vi "HEWH Adjust Temp Flow.vi"(0 "Core HEWH Data Station A":T2 {"Test Patten Setup"."PRAT/RLT Sequence"."Time" format="%<%H:%M:%S>t"; "Test Patten Setup"."Total Gallons Schedule" format="%.2f"}, 1 "MW100 Input":refnum<visa-resource-name>, 2 "Disable Temp Adjust?":bool, 3 "MW100 Sema":T18, 4 "GPM Target":T19 format="%.2f", 5 "error in (no error)":errorcluster, 6 "Elapsed Time (sec)":dbl, 7 "Temperature":T19 format="%.2f", 8 "State":T1, 10 "PID gains (Temp)":T20={"proportional gain (Kc)"=0.1, "integral time (Ti, min)"=0.01, "derivative time (Td, min)"=0.0} {"derivative time (Td, min)" format="%.3f"; "integral time (Ti, min)" format="%.3f"; "proportional gain (Kc)" format="%.3f"}, 11 "Debug":bool, 12 "Adjust Temp Timer":dbl=1.0 format="%#_13g", 13 "Use Fuzzy Logic":bool) -> (14 "Core HEWH Data out":T2 {"Test Patten Setup"."PRAT/RLT Sequence"."Time" format="%<%H:%M:%S>t"; "Test Patten Setup"."Total Gallons Schedule" format="%.2f"}, 15 "MW100 Output":refnum<visa-resource-name>, 18 "Adjusting Temp":bool, 19 "error out":errorcluster)   [LabVIEW 2016]
uses:
  Utility/Custom Pallet Controls/Custom Pallet DBL.ctl
  Type Definitions/HEWH Output Information.ctl
  Type Definitions/HEWH Draw Pattern Setup.ctl
  Type Definitions/PRAT Test.ctl
  Utility/Save File/File Setup (Public)/Type Definition/Save File HEWH Heating Control Mode.ctl
  Type Definitions/Terminate Draw Conditions.ctl
  Type Definitions/HEWH Start Conditions.ctl
  Type Definitions/Check Special Condtions.ctl
  Type Definitions/HEWH Special Condition Check.ctl
  Type Definitions/HEWH Draw Flag ENUM.ctl
  Type Definitions/HEWH Specific DAQ.ctl
  Type Definitions/HEWH Power Data.ctl
  Type Definitions/HEWH Power Elements.ctl
  Utility/Type Definitions/UTILITY Power Analyzer.ctl
  Type Definitions/HEWH Calc and Calibration.ctl
  Utility/Save File/File Setup (Public)/Type Definition/Save File DOE LabView Program.ctl
  Custom Instrument Control/MW100/Type Definitions/Station ID Selector.ctl
  Type Definitions/HEWH Purge Draw.ctl
  Utility/Save File/File Setup.lvlib
panel:
  out "uA Output Flow":i32
  out "uA Output Temp":i32
  # "Draw Pattern Setup (24 Hour)"
  # "Draw Pattern Setup (24 Hour)"
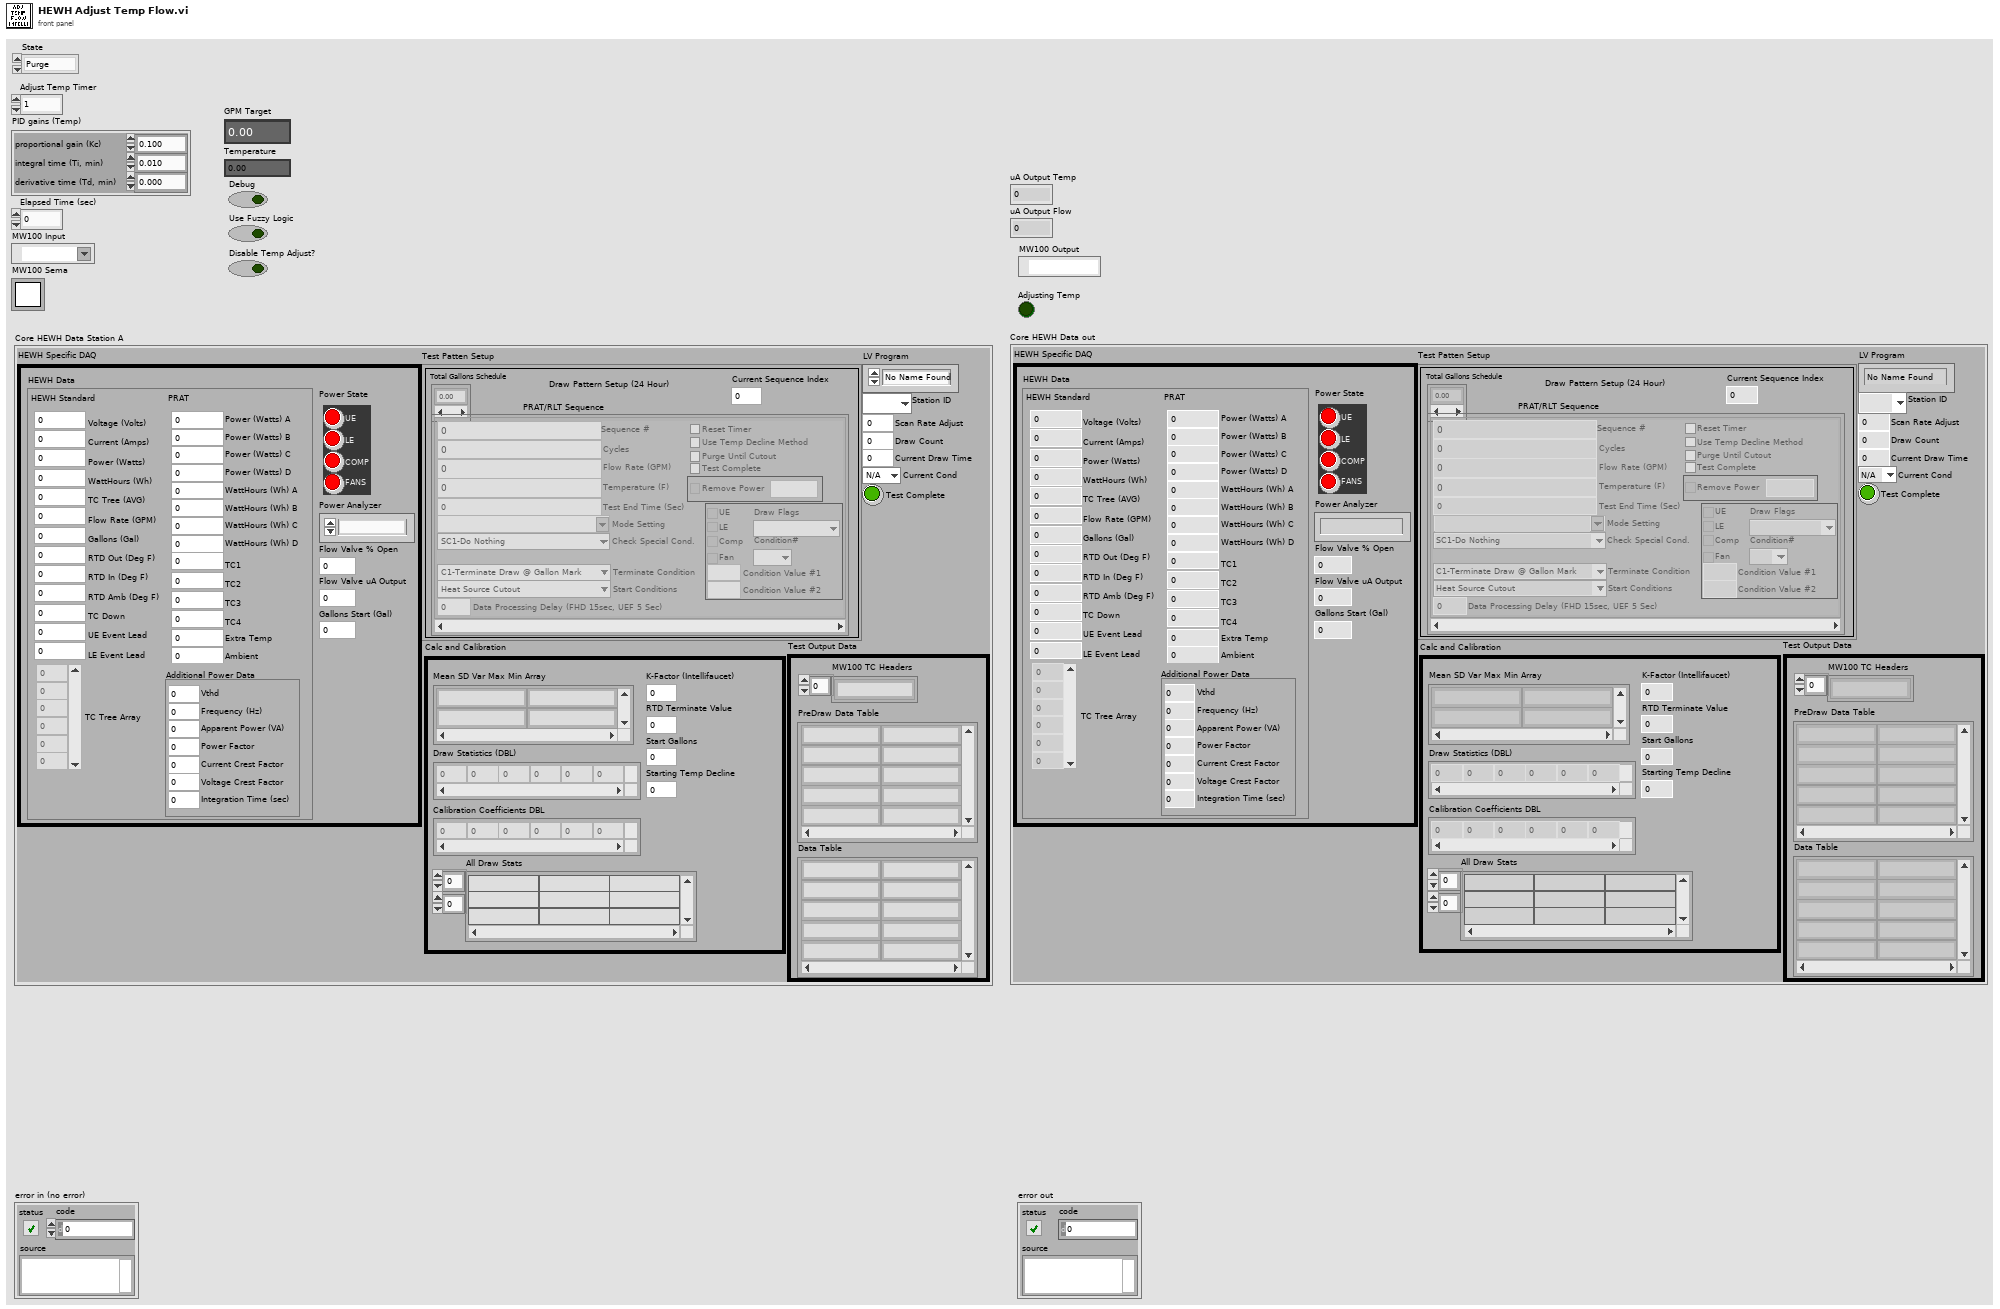
[diagram p1: front panel]
types:
  T1 = typedef "HEWH Purge Draw.ctl" = enum16{"Purge", "Draw"}
  T2 = typedef "HEWH Output Information.ctl" = cluster{"Scan Rate Adjust":dbl, "Draw Count":i32, "Test Patten Setup":T3, "HEWH Specific DAQ":T11, "Test Output Data":cluster{"PreDraw Data Table":string[][], "Data Table":string[][], "MW100 TC Headers":string[]}, "Calc and Calibration":T15, "Current Draw Time":dbl, "LV Program":T16, "Station ID":T17, "Current Cond":T9, "Test Complete":bool}
  T3 = typedef "HEWH Draw Pattern Setup.ctl" = cluster{"Total Gallons Schedule":dbl[], "PRAT/RLT Sequence":T4[], "Current Sequence Index":i32}
  T4 = typedef "PRAT Test.ctl" = cluster{"Sequence #":dbl, "Cycles":i32, "Mode Setting":T5, "Flow Rate (GPM)":dbl, "Temperature (F)":dbl, "Reset Timer":bool, "Use Temp Decline Method":bool, "Terminate Condition":T6, "Condition Value #1":dbl, "UE":bool, "LE":bool, "Comp":bool, "Fan":bool, "Test End Time (Sec)":dbl, "Purge Until Cutout":bool, "Start Conditions":T7, "Condition Value #2":dbl, "Remove Power":bool, "Time":dbl, "Check Special Cond.":T8, "Condition#":T9, "Draw Flags":T10, "Data Processing Delay (FHD 15sec, UEF 5 Sec)":dbl, "Test Complete":bool}
  T5 = typedef "File Setup.lvlib/Save File HEWH Heating Control Mode.ctl" = string
  T6 = typedef "Terminate Draw Conditions.ctl" = enum16{"C1-Terminate Draw @ Gallon Mark", "C2-Special Last Draw (HU Test)", "C3-RTD Out <=", "C4-Mean Tank Temp <=", "C5-Decrease RTD Out (Deg F)", "C6-Time (Seconds)", "C7-Until Any Heat Source", "C8-Specific Heat Source", "C9-Do Nothing"}
  T7 = typedef "HEWH Start Conditions.ctl" = enum16{"Heat Source Cutout", "At Time (Seconds)", "Every X (Seconds)", "T2 >= X° Below Setpoint", "Seconds From Complete", "Wait for LE & Comp Cutout", "Wait for Comp Cutout", "Wait for LE Cutout", "Wait for UE Cutout"}
  T8 = typedef "Check Special Condtions.ctl" = enum16{"SC1-Do Nothing", "SC2-Check Heat Source (On-C2/Off-C1)", "SC3-Check Skip Condition", "SC4-Check Heat Source ON/Fail"}
  T9 = typedef "HEWH Special Condition Check.ctl" = enum16{"N/A", "C1", "C2", "Reset/Fail", "Skip Draw Sequence"}
  T10 = typedef "HEWH Draw Flag ENUM.ctl" = enum16{"N/A", "None(0)", "Sml(1)", "Med(2)", "SmlMed(3)", "Lrg(4)", "SmlLrg(5)", "MedLrg(6)", "SmlMedLrg(7)"}
  T11 = typedef "HEWH Specific DAQ.ctl" = cluster{"HEWH Data":T12, "Flow Valve % Open":dbl, "Power State":T13, "Power Analyzer":T14, "Flow Valve uA Output":i32, "Gallons Start (Gal)":dbl}
  T12 = typedef "HEWH Power Data.ctl" = cluster{"HEWH Standard":cluster{"Voltage (Volts)":dbl, "Current (Amps)":dbl, "Power (Watts)":dbl, "WattHours (Wh)":dbl, "TC Tree (AVG)":dbl, "Flow Rate (GPM)":dbl, "Gallons (Gal)":dbl, "RTD Out (Deg F)":dbl, "RTD In (Deg F)":dbl, "RTD Amb (Deg F)":dbl, "TC Down":dbl, "UE Event Lead":i32, "LE Event Lead":i32, "TC Tree Array":dbl[]}, "PRAT":cluster{"Power (Watts) A":dbl, "Power (Watts) B":dbl, "Power (Watts) C":dbl, "Power (Watts) D":dbl, "TC1":dbl, "TC2":dbl, "TC3":dbl, "TC4":dbl, "WattHours (Wh) A":dbl, "WattHours (Wh) B":dbl, "WattHours (Wh) C":dbl, "WattHours (Wh) D":dbl, "Ambient":dbl, "Extra Temp":dbl}, "Additional Power Data":cluster{"Vthd":dbl, "Frequency (Hz)":dbl, "Apparent Power (VA)":dbl, "Power Factor":dbl, "Current Crest Factor":dbl, "Voltage Crest Factor":dbl, "Integration Time (sec)":dbl}}
  T13 = typedef "HEWH Power Elements.ctl" = cluster{"UE":bool, "LE":bool, "COMP":bool, "FANS":bool}
  T14 = typedef "UTILITY Power Analyzer.ctl" = enum16{"", "APLUS", "WT210", "WT500", "WT300", "OSI", "Debug", "WT230", "WT300_1", "WT300_2"}
  T15 = typedef "HEWH Calc and Calibration.ctl" = cluster{"Mean SD Var Max Min Array":string[][], "Draw Statistics (DBL)":dbl[][], "Calibration Coefficients DBL":dbl[][], "Start Gallons":dbl, "Starting Temp Decline":dbl, "K-Factor (Intellifaucet)":dbl, "All Draw Stats":string[][], "RTD Terminate Value":dbl}
  T16 = typedef "File Setup.lvlib/Save File DOE LabView Program.ctl" = enum16{"No Name Found", "DOE Stand", "Dishwasher Kitchen", "Portable Stand", "HEWH", "Dryer", "Dryer WILT", "HCC", "PRAT", "HEWH RLT", "Refrigeration"}
  T17 = typedef "Station ID Selector.ctl" = enum16{"", "A", "B", "C", "D", "Global"}
  T18 = typedef "Semaphore RefNum" = refnum<k1>
  T19 = typedef "Custom Pallet DBL.ctl" = dbl
  T20 = cluster{"proportional gain (Kc)":dbl, "integral time (Ti, min)":dbl, "derivative time (Td, min)":dbl}
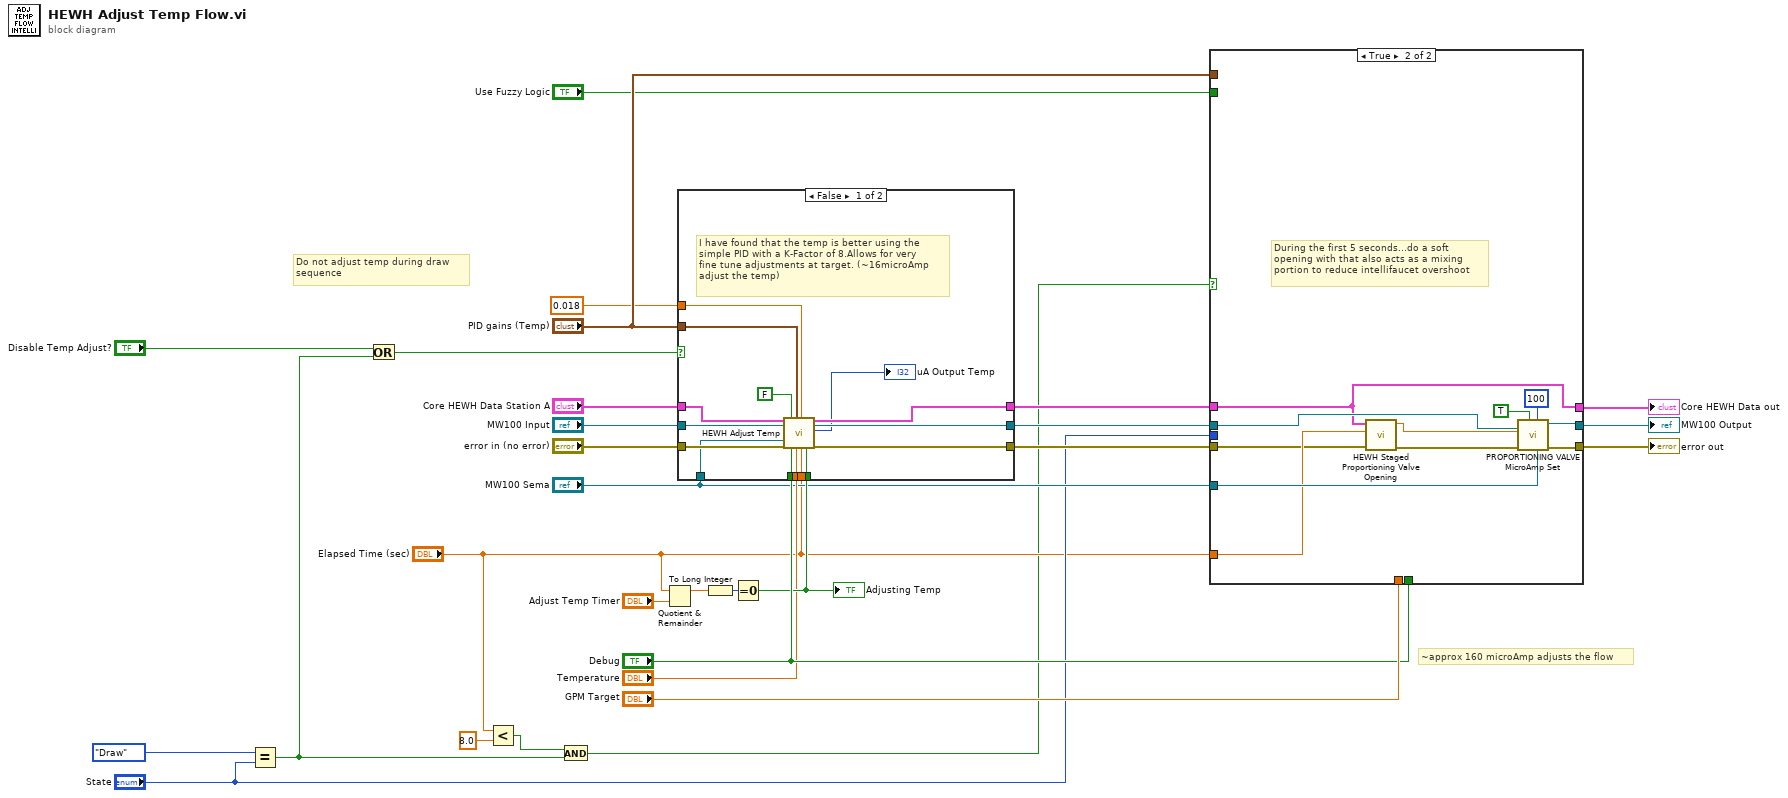
[diagram p0: block diagram]
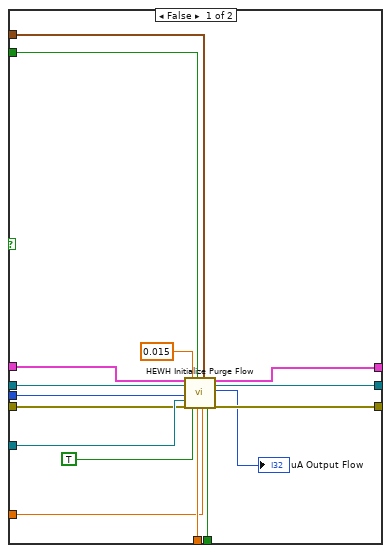
[diagram p3: hidden frame]
diagram:
  # "Do not adjust temp during draw \nsequence"
  # "~approx 160 microAmp adjusts the flow"
  n1 = Equal?(x=HEWH_Purge_Draw."Draw", y="State") -> (x = y?=w2:bool)
  n2 = Or(x="Disable Temp Adjust?", y=w2) -> (x .or. y?=w6:bool)
  n3 = Less?(x="Elapsed Time (sec)", y=8.0) -> (x < y?=w3:bool)
  n4 = And(x=w3, y=w2) -> (x .and. y?=w1:bool)
  n5 = Quotient & Remainder(x="Elapsed Time (sec)", y="Adjust Temp Timer") -> (x-y*floor(x/y)=w22:dbl)  [unwired: 1 out]
  n6 = To Long Integer(number=w22) -> (32bit integer=w21:i32)
  n7 = Equal To 0?(x=w21) -> (x = 0?=w24:bool)
  "Adjusting Temp" <- w24
  n8 = case shown="False" w6 {
    tunnel: "Debug" -> [w44 _]
    tunnel: "PID gains (Temp)" -> [w43 _]
    tunnel: w24 -> [w42 _]
    tunnel: [w41 w47] -> w20
    tunnel: "Core HEWH Data Station A" -> [w40 w47]
    tunnel: [w39 w46] -> w18
    tunnel: "error in (no error)" -> [w38 w45]
    tunnel: "MW100 Input" -> [w37 w46]
    tunnel: "Temperature" -> [w36 _]
    tunnel: 0.018 ("ErrorPassBand(%)") -> [w35 _]
    tunnel: [w34 w45] -> w12
    tunnel: "MW100 Sema" -> [w31 _]
    tunnel: "Elapsed Time (sec)" -> [w30 _]
    frame False {
      # "I have found that the temp is better using the\nsimple PID with a K-Factor of 8.Allows for very\nfine tune adjustments at target. (~16microAmp\nadjust the temp)"
      n9 = call "HEWH Adjust Temp.vi"("Core HEWH Data Input"=w40, "MW100"=w37, "MW100 Sema"=w31, "error in (no error)"=w38, "Use Fuzzy Logic"=FALSE, "Debug"=w44, "PID gains"=w43, "Temperature"=w36, "ErrorPassBand(%)"=w35, "Elapsed Time (sec)"=w30, "Adjust Temp"=w42) -> ("Core HEWH Data Output"=w41:T2, "MW100 Out"=w39:refnum<visa-resource-name>, "uA Output"=→"uA Output Temp":i32, "error out"=w34:errorcluster)  [unwired: 5 in]
    }
    frame True {
    }
  }
  n10 = case shown="True" w1 {
    tunnel: "GPM Target" -> [w63 _]
    tunnel: "Debug" -> [w62 _]
    tunnel: [w61 w72] -> w27
    tunnel: [w60 w69] -> w26
    tunnel: "PID gains (Temp)" -> [w59 _]
    tunnel: "MW100 Sema" -> [w58 w68]
    tunnel: w20 -> [w57 w69]
    tunnel: w18 -> [w56 w71]
    tunnel: [w55 w70] -> w15
    tunnel: w12 -> [w52 w66]
    tunnel: "Use Fuzzy Logic" -> [w50 _]
    tunnel: "State" -> [w49 _]
    tunnel: "Elapsed Time (sec)" -> [w48 w67]
    frame False {
      n11 = call "HEWH Initialize Purge Flow.vi"("Core HEWH Data in"=w57, "MW100"=w56, "State"=w49, "MW100 Sema"=w58, "error in (no error)"=w52, "ErrorPassBand(%)"=0.015, "Use Proportion Valve"=TRUE, "Use Fuzzy Logic"=w50, "GPM Target"=w63, "PID gains"=w59, "Elapsed Time (sec)"=w48, "Debug"=w62) -> ("Core HEWH Data out"=w60:T2, "MW100 Out"=w55:refnum<visa-resource-name>, "uA Output"=→"uA Output Flow":i32, "error out"=w61:errorcluster)  [unwired: 4 in]
    }
    frame True {
      # "During the first 5 seconds...do a soft\nopening with that also acts as a mixing \nportion to reduce intellifaucet overshoot"
      n12 = call "HEWH Staged Proportioning Valve Opening.vi"("Error In"=w66, "Elapsed Time (sec) in"=w67, "Core HEWH Data Station A"=w69) -> ("Error Out"=w65:errorcluster, "Prop Valve Setting"=w64:dbl)  [unwired: 7 in]
      n13 = call "PROPORTIONING VALVE MicroAmp Set.vi"("Refnum in"=w68, "milliseconds to wait"=u32 100, "Use Micro Amp Set"=TRUE, "error in (no error)"=w65, "Target"=w64, "VISA Refnum in"=w71) -> ("error out"=w72:errorcluster, "VISA Refnum out"=w70:refnum<visa-resource-name>)  [unwired: 4 in]
    }
  }
  "error out" <- w27
  "Core HEWH Data out" <- w26
  "MW100 Output" <- w15
